vi "Set AOD Scanning Offsets.vi"(6 "Scan Settings":T1, 7 "Scan Settings (um)":T1={"XStart"=-100, "XEnd"=100, "XNum"=250, "YStart"=-100, "YEnd"=100, "YNum"=250, "ZStart"=-30, "ZEnd"=70, "ZNum"=60}, 8 "Scan Offset Z":dbl format="%#_13g", 9 "Scan Offset Y":dbl format="%#_13g", 10 "Scan Offset X":dbl format="%#_13g", 11 "FPGA VI Reference":T2) -> ()   [LabVIEW 2014]
uses:
  FPGA_Control/AODRef.ctl
  <vilib>/Utility/error.llb/Error Cluster From Error Code.vi
  <vilib>/rvi/errors/niLvFpgaAdjustHostInterfaceError.vi
  <vilib>/rvi/interface/nirviReadWriteControl/nirviReadWriteControl.xnode
  FPGA Bitfiles/AodScanner_FPGATarget_AODControl(FPGA)_TyJc9yYmyGA.lvbitx
  NiFpgaLv.dll
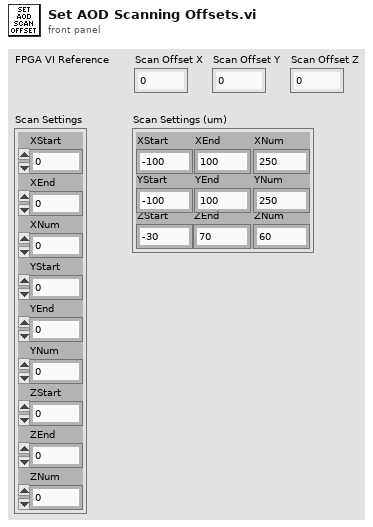
[diagram p1: front panel]
types:
  T1 = cluster{"XStart":i32, "XEnd":i32, "XNum":i32, "YStart":i32, "YEnd":i32, "YNum":i32, "ZStart":i32, "ZEnd":i32, "ZNum":i32}
  T2 = typedef "AODRef.ctl" = refnum<k20>
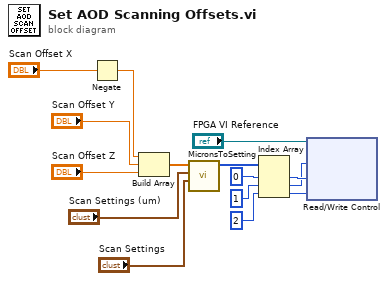
[diagram p0: block diagram]
diagram:
  n1 = Negate(x="Scan Offset X") -> (-x=w1:dbl)
  n2 = Build Array(w1, "Scan Offset Y", "Scan Offset Z") -> (w8:dbl[])
  n3 = call "MicronsToSetting.vi"("Scan Settings"="Scan Settings", "Scan Settings (um)"="Scan Settings (um)", "Microns (X,Y,Z)"=w8) -> ("Setting"=w12:i32[])  [unwired: 8 in]
  n4 = Index Array(array=w12, index #1=0 ("index"), index #2=1 ("index"), index #3=2 ("index")) -> (element #1=w7:i32, element #2=w6:i32, element #3=w11:i32)
  n5 = xnode "Read/Write Control"("FPGA VI Reference In"="FPGA VI Reference", "InOffset.X"=w6, "InOffset.Y"=w7, "InOffset.Z"=w11) -> ()  [unwired: 1 in, 2 out]
